vi "MyTest.vi"() -> ()   [LabVIEW 2024]
panel:
  in  "Gmax":dbl
  in  "Gmin":dbl
  in  "Gavg":dbl
  in  "Calculate":bool
  in  "Read RB 2":bool
  in  "Read RB":bool
  in  "B":dbl
  out "?":bool
  out "RG":dbl[](array[numeric]) caption="RB" format="%_6f"
  out "RB":dbl[](array[numeric]) format="%_6f"
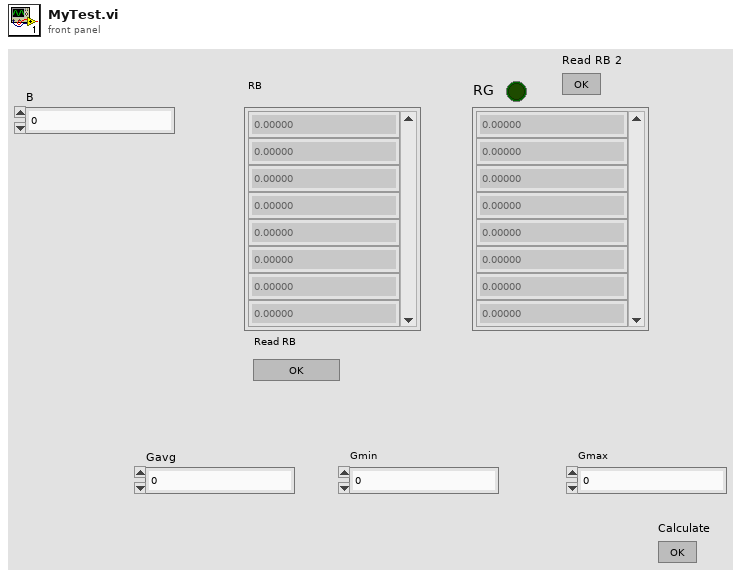
[diagram p1: front panel]
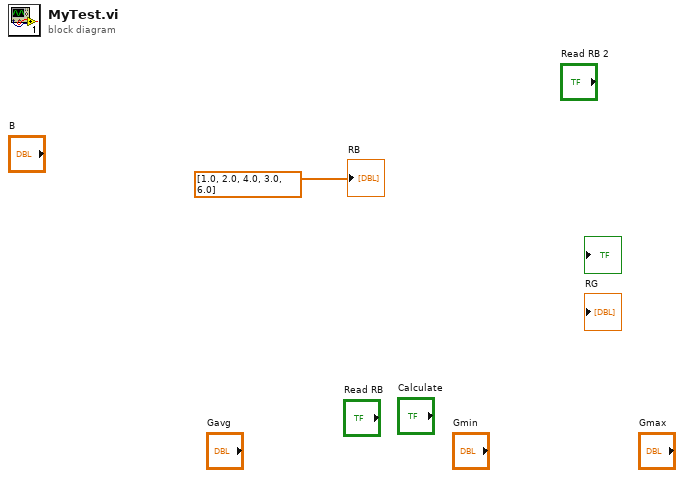
[diagram p0: block diagram]
diagram:
  "RB" <- dbl[] [1.0, 2.0, 4.0, 3.0, 6.0] ("RB")
